vi "Copy Template.vi"(11 "error in (no error)":errorcluster) -> (15 "error out":errorcluster)   [LabVIEW 2021, in "G Plug-in Migrator.lvlib"]
uses:
  G Plug-in Migrator.lvlib
  _Editor/controls/Data Holder.ctl
  _Editor/G-Plugin Editor.lvlib
  Migrator Reusables/Migrator Reusables.lvlib
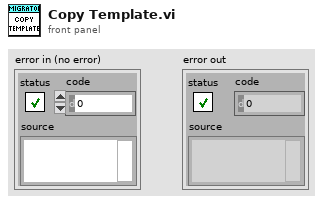
[diagram p1: front panel]
types:
  T1 = typedef "G-Plugin Editor.lvlib/Data Holder.ctl" = cluster{"project ref":refnum<vi>, "Name":string, "Plugin Type":string, "Plugin Group Name":string}
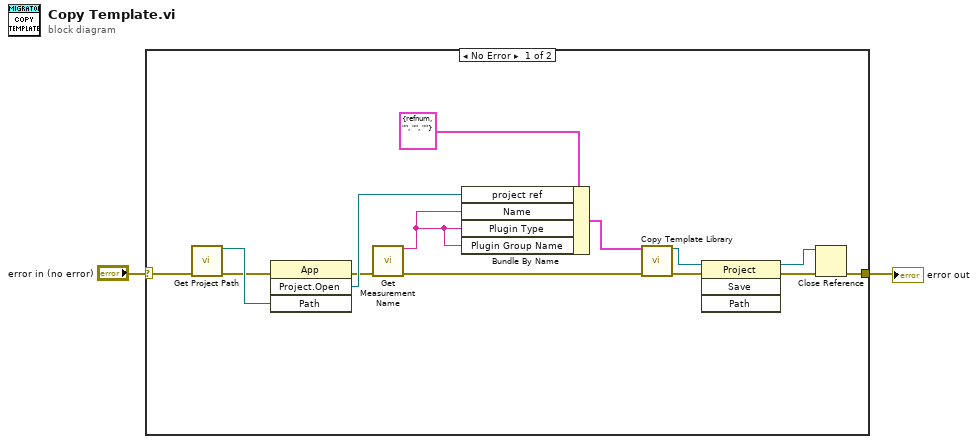
[diagram p0: block diagram]
diagram:
  n1 = case shown="No Error" "error in (no error)" {
    selector: "error in (no error)" -> [w13 w17]
    tunnel: [w4 w17] -> w2
    frame No Error {
      n2 = call "Get Project Path.vi"("error in (no error)"=w13) -> ("Project Path Out"=w15:path, "error out"=w14:errorcluster)  [unwired: 13 in]
      n3 = invoke class="App" method="Project.Open"(error in=w14, "Path"=w15) -> (error out=w9:errorcluster, "Project:Open"=w11:refnum<vi>)  [unwired: 2 in, 2 out]
      n4 = call "Get Measurement Name.vi"("error in (no error)"=w9) -> ("Name Out"=w8:string, "error out"=w10:errorcluster)  [unwired: 13 in]
      n5 = Bundle By Name(cluster=T1 {"project ref"=refnum, "Name"="", "Plugin Type"="", "Plugin Group Name"=""} ("Configuration"), "project ref"=w11, "Name"=w8, "Plugin Type"=w8, "Plugin Group Name"=w8) -> (w12:T1)
      n6 = call "Copy Template Library.vi"("Configuration"=w12, "error in (no error)"=w10) -> ("project ref out"=w7:refnum<vi>, "error out"=w6:errorcluster)  [unwired: 12 in]
      n7 = invoke class="Project" method="Save"(reference=w7, error in=w6) -> (reference out=w3:refnum<vi>, error out=w5:errorcluster)  [unwired: 2 in, 2 out]
      n8 = Close Reference(reference=w3, error in (no error)=w5) -> (error out=w4:errorcluster)
    }
    frame Error {
    }
  }
  "error out" <- w2
